vi "2a_ths_browser_mpix.vi"() -> ()   [LabVIEW 2021]
panel:
  in  "file (use dialog)":path=path "C:/scan/thscan.bin"
  out "MainImg":u16[][](graph)
  out "Th Scan":u16[](graph)
  in  "ThScan_Load":bool
  out "ThScan":i32[][][](array[numeric])
  in  "Exit":bool
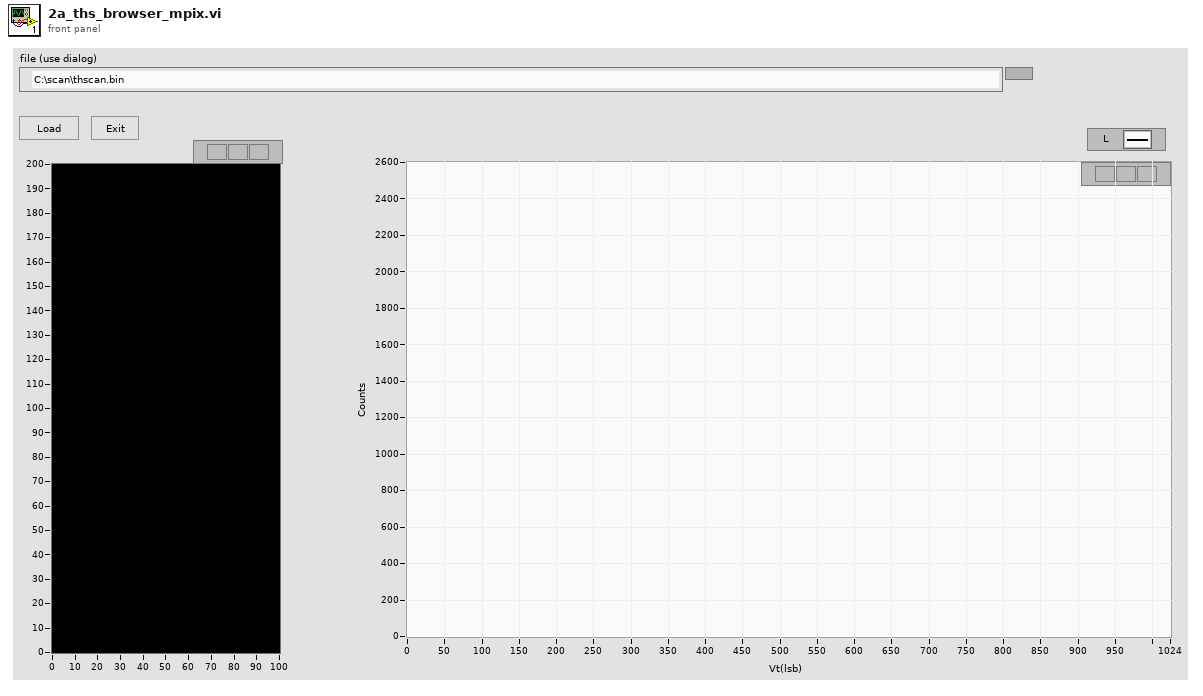
[diagram p1: front panel]
types:
  T1 = enum16{"big-endian, network order", "native, host order", "little-endian"}
  T2 = typedef "LVPointDoubleTypeDef.ctl" = cluster{"Cursor X":dbl, "Cursor Y":dbl}
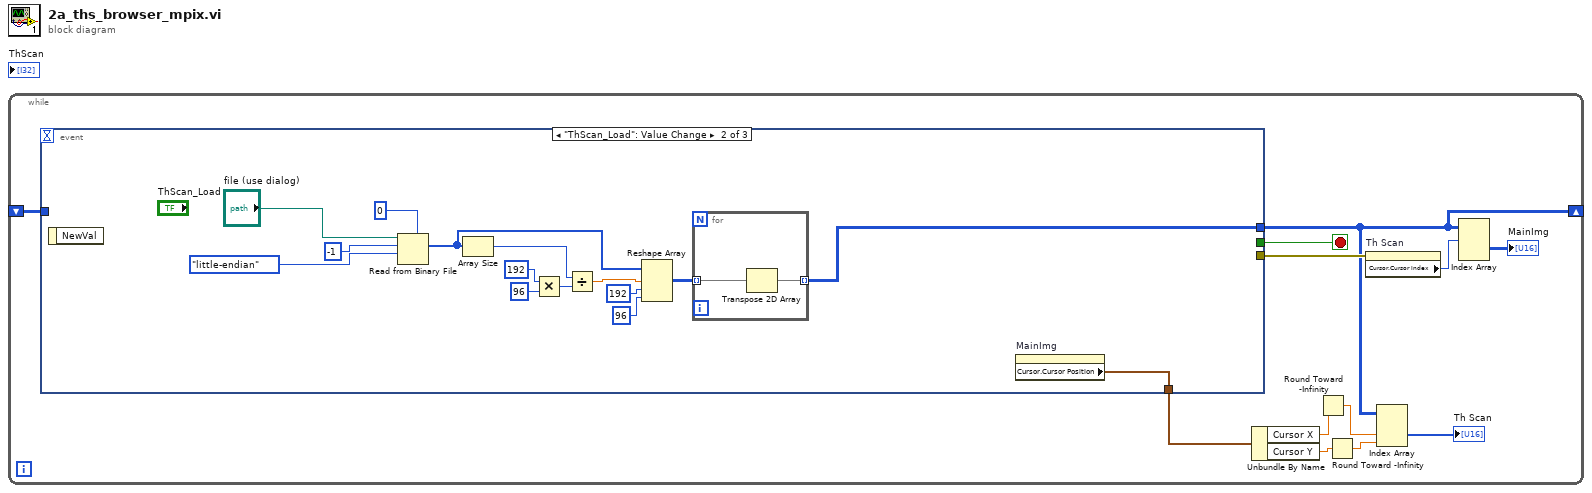
[diagram p0: block diagram]
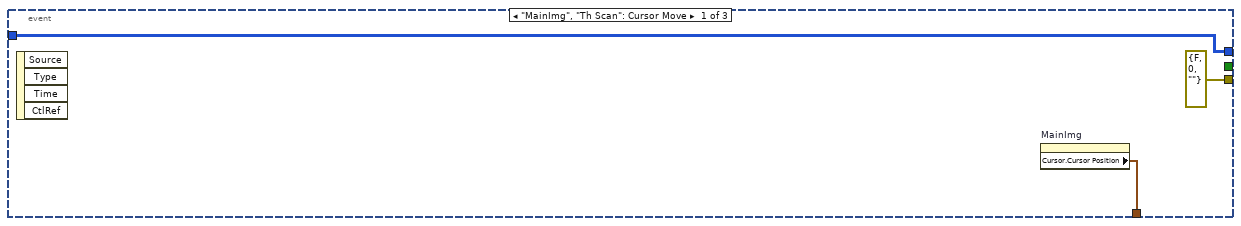
[diagram p2: hidden frame]
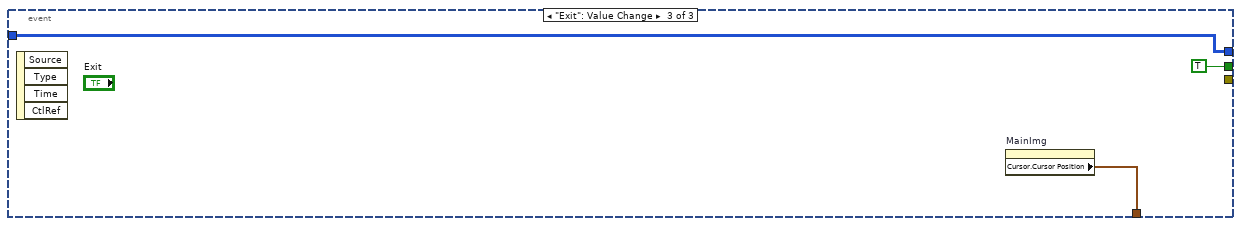
[diagram p3: hidden frame]
diagram:
  n1 = while {
    shift-right: [w7] -> _
    shift-left: _ -> [w6]
    stop <- w12 stop-if-true
    n2 = event shown="[1] \"ThScan_Load\": Value Change" {
      selector: _ -> [_ _ _]
      dyn-events: _ -> [_ _ _]
      timeout: _ -> [_ _ _]
      tunnel: [_ _ TRUE] -> w12
      tunnel: [errorcluster {"status"=FALSE, "code"=0, "source"=""} ("error in (no error)") _ _] -> w8
      tunnel: w6 -> [w14 _ w34]
      tunnel: [w14 w30 w34] -> w7
      tunnel: [w13 w29 w33] -> w3
      event "MainImg", "Th Scan": Cursor Move {
        n3 = event-data() -> ()  [unwired: 1 in, 4 out]
        n4 = property on="MainImg" class="IntGraph (strict)"() -> ("Cursor.Cursor Position"=w13:T2)  [unwired: 2 in, 2 out]
      }
      event "ThScan_Load": Value Change {
        n5 = event-data() -> ()  [unwired: 1 in, 1 out]
        n6 = Read from Binary File(5:u16 0, 9:T1."little-endian" ("byte order (0:big-endian, network order)"), 10:-1 ("count (1)"), 11:"file (use dialog)") -> (2:w17:u16[])  [unwired: 2 in, 3 out]
        n7 = Array Size(array=w17) -> (size(s)=w22:i32)
        n8 = Multiply(x=192 ("dimension size"), y=96 ("dimension size")) -> (x*y=w19:i32)
        n9 = Divide(x=w22, y=w19) -> (x/y=w18:dbl)
        n10 = Reshape Array(w17, w18, 192 ("dimension size"), 96 ("dimension size")) -> (w16:u16[][][])
        n11 = for {
          tunnel: w16 -> [w32] mode=indexing
          tunnel: [w31] -> w30 mode=indexing
          n12 = Transpose 2D Array(2D array=w32) -> (transposed array=w31:u16[][])
        }
        n13 = property on="MainImg" class="IntGraph (strict)"() -> ("Cursor.Cursor Position"=w29:T2)  [unwired: 2 in, 2 out]
      }
      event "Exit": Value Change {
        n14 = event-data() -> ()  [unwired: 1 in, 4 out]
        n15 = property on="MainImg" class="IntGraph (strict)"() -> ("Cursor.Cursor Position"=w33:T2)  [unwired: 2 in, 2 out]
      }
    }
    n16 = Unbundle By Name(w3) -> ("Cursor X"=w2:dbl, "Cursor Y"=w4:dbl)
    n17 = Round Toward -Infinity(1:w2) -> (0:w1:dbl)
    n18 = Round Toward -Infinity(1:w4) -> (0:w5:dbl)
    n19 = property on="Th Scan" class="WFGraph (strict)"(error in=w8) -> ("Cursor.Cursor Index"=w9:i32)  [unwired: 1 in, 2 out]
    n20 = Index Array(array=w7, index (dim 1)=w1, index (dim 2)=w5) -> (element=→"Th Scan":u16[])  [unwired: 1 in]
    n21 = Index Array(array=w7, index (dim 0)=w9) -> (element=→"MainImg":u16[][])  [unwired: 2 in]
  }
